vi "Scanning.vi"() -> ()   [LabVIEW 2017]
uses:
  <vilib>/measure/mascope.llb/Amplitude and Levels N chan.vi
  <vilib>/Utility/file.llb/Write Delimited Spreadsheet (DBL).vi
  <vilib>/measure/NI_MABase.lvlib
  <vilib>/measure/NI_MAPro.lvlib
  <vilib>/Analysis/NI_AALBase.lvlib
panel:
  in  "Save?":bool
  out "Mini":dbl=-8.956477094616275
  out "VISIBILITY":dbl=0.98937154039023
  in  "BG":dbl=-9.0489
  in  "Position":string="Align_MZ5"
  out "Amplitude vs Path difference":T1(graph)={"median"=17.205295164807467, "median"=8.246886175271356, "median"=-8.957926015806152}
  in  "Folder":path=path "C:/Users/Weak/Desktop/September/BD_CV_MH_MZ/Alignment"
  out "Scanning":dynamicdata(graph)=[{"t0"=timestamp(3620982824.2666583 s since 1904-01-01), "dt"=1.9999999999999998e-05, "Y"=array[5000 elements], "attributes"=variant("NI_ChannelName"=variant(string "Voltage_0"), "NI_UnitDescription"=variant(string "Volts"))}, {"t0"=timestamp(3620982824.2666683 s since 1904-01-01), "dt"=1.9999999999999998e-05, "Y"=array[5000 elements], "attributes"=variant("NI_ChannelName"=variant(string "Voltage_1"), "NI_UnitDescription"=variant(string "Volts"))}]
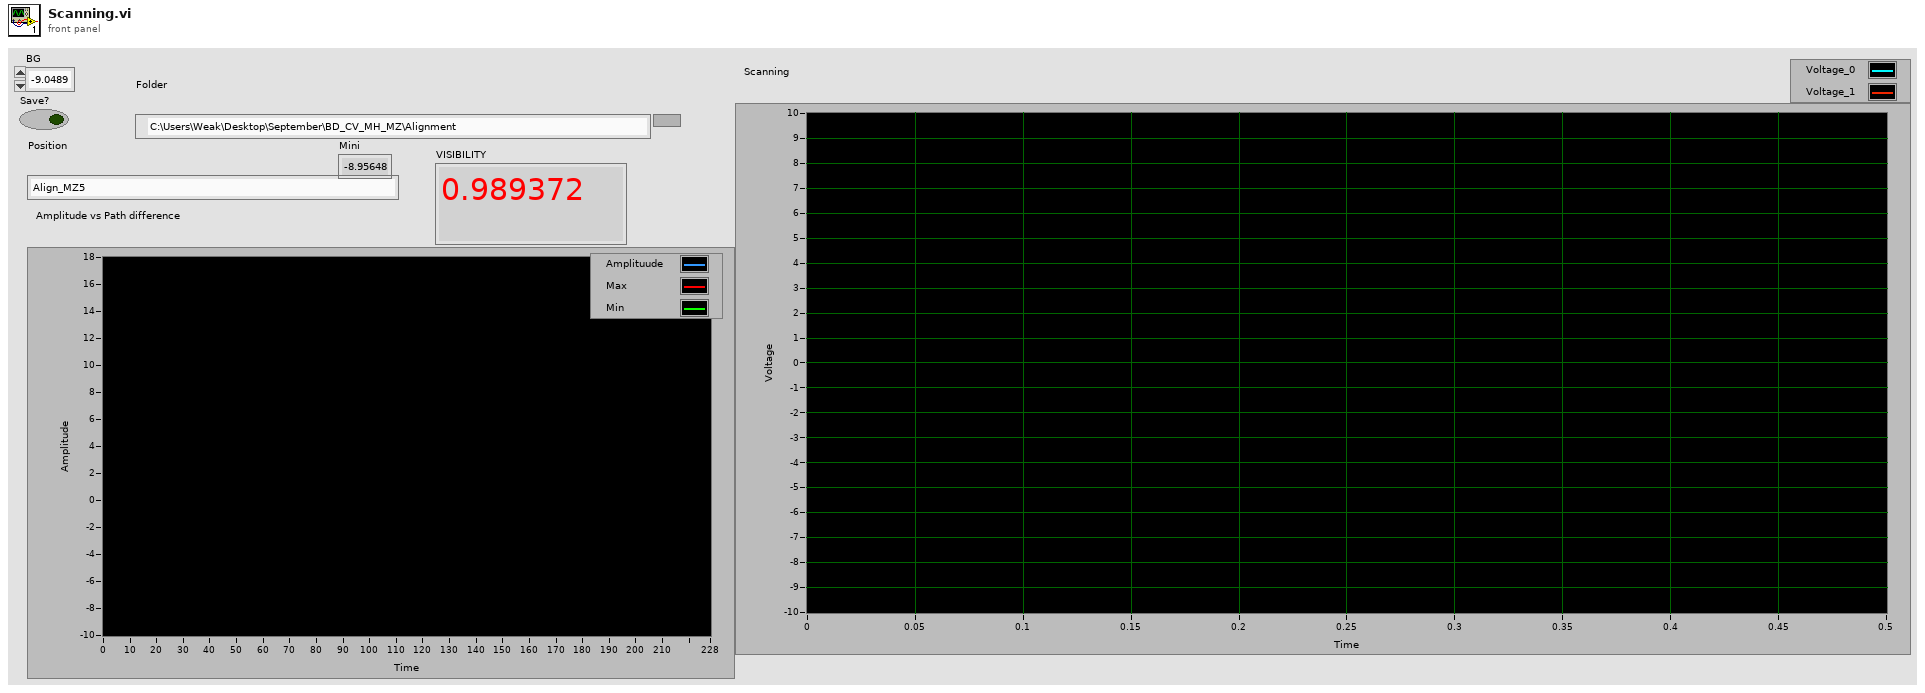
[diagram p1: front panel]
types:
  T1 = cluster{"median":dbl, "median":dbl, "median":dbl}
  T2 = enum16{"Sine Wave", "Triangle Wave", "Square Wave", "Sawtooth Wave"}
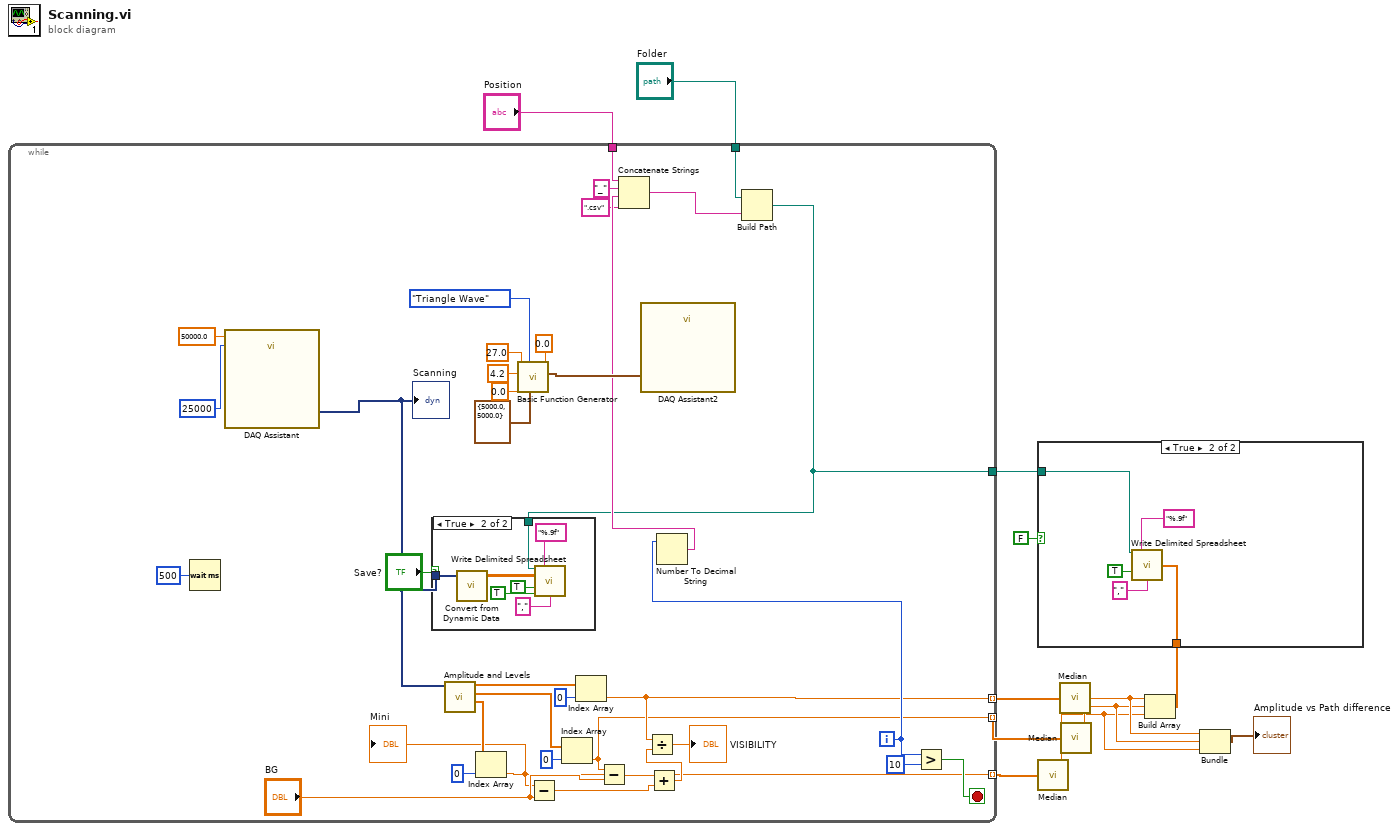
[diagram p0: block diagram]
diagram:
  n1 = while {
    tunnel: "Folder" -> [w34]
    tunnel: "Position" -> [w32]
    tunnel: [w21] -> w10 mode=indexing
    tunnel: [w15] -> w9 mode=indexing
    tunnel: [w14] -> w8 mode=indexing
    tunnel: [w13] -> w3
    i -> [w30]
    stop <- w35 stop-if-true
    n2 = Wait (ms)(milliseconds to wait=u32 500) -> ()  [unwired: 1 out]
    n3 = call "DAQ Assistant"("rate"=50000.0, "number of samples"=25000) -> ("data"=w39:dynamicdata)  [unwired: 15 in, 2 out]
    "Scanning" <- w39
    n4 = call-poly <vilib>:"Amplitude and Levels.vi"("signal(s) in"=w39) -> ("low state level"=w23:dbl[], "high state level"=w25:dbl[], "amplitude"=w38:dbl[])  [unwired: 7 in, 1 out]
    n5 = Index Array(array=w23, index=0) -> (element=w14:dbl)
    "Mini" <- w14
    n6 = call <vilib>:"Basic Function Generator.vi"("offset"=0.0, "sampling info"=cluster{"Fs":dbl, "#s":dbl} {"Fs"=5000.0, "#s"=5000.0}, "signal type"=T2."Triangle Wave", "phase"=0.0, "amplitude"=4.2, "frequency"=27.0) -> ("signal out"=w40:waveform(dbl))  [unwired: 3 in, 2 out]
    n7 = Subtract(x=w14, y="BG") -> (x-y=w19:dbl)
    n8 = Index Array(array=w25, index=0) -> (element=w15:dbl)
    n9 = Index Array(array=w38, index=0) -> (element=w21:dbl)
    n10 = Subtract(x=w15, y="BG") -> (x-y=w20:dbl)
    n11 = call "DAQ Assistant2"("data"=w40) -> ()  [unwired: 17 in, 2 out]
    n12 = Add(x=w20, y=w19) -> (x+y=w18:dbl)
    n13 = Divide(x=w21, y=w18) -> (x/y=→"VISIBILITY":dbl)
    n14 = Number To Decimal String(number=w30) -> (decimal integer string=w29:string)  [unwired: 1 in]
    n15 = Concatenate Strings(w32, "_" ("string"), w29, ".csv" ("string")) -> (w33:string)
    n16 = Build Path(base path=w34, name or relative path=w33) -> (appended path=w13:path)
    n17 = case shown="True" "Save?" {
      tunnel: w39 -> [_ w52]
      tunnel: w13 -> [_ w51]
      frame False {
      }
      frame True {
        n18 = call "Convert from Dynamic Data"("Dynamic Data Type"=w52) -> ("Array"=w49:dbl[][])  [unwired: 3 in]
        n19 = call-poly <vilib>:"Write Delimited Spreadsheet.vi"("file path (dialog if empty)"=w51, "format (%.3f)"="%.9f", "2D data"=w49, "append to file? (new file:F)"=TRUE, "transpose? (no:F)"=TRUE, "delimiter (\\t)"="," ("delimiter (\\t)")) -> ()  [unwired: 8 in, 2 out]
      }
    }
    n20 = Greater?(x=w30, y=10) -> (0:w35:bool)
  }
  n21 = call <vilib>:"Median.vi"("X"=w8) -> ("median"=w5:dbl)  [unwired: 1 out]
  n22 = call <vilib>:"Median.vi"("X"=w10) -> ("median"=w7:dbl)  [unwired: 1 out]
  n23 = call <vilib>:"Median.vi"("X"=w9) -> ("median"=w6:dbl)  [unwired: 1 out]
  n24 = Build Array(w7, w6, w5) -> (w2:dbl[])
  n25 = case shown="True" FALSE {
    tunnel: w3 -> [_ w58]
    tunnel: w2 -> [_ w56]
    frame False {
    }
    frame True {
      n26 = call-poly <vilib>:"Write Delimited Spreadsheet.vi"("file path (dialog if empty)"=w58, "format (%.3f)"="%.9f", "1D data"=w56, "append to file? (new file:F)"=TRUE, "delimiter (\\t)"="," ("delimiter (\\t)")) -> ()  [unwired: 9 in, 2 out]
    }
  }
  n27 = Bundle("median"=w7, "median"=w6, "median"=w5) -> (→"Amplitude vs Path difference":T1)  [unwired: 1 in]
